vi "Debug Server First Launch.vi"(8 "error in (no error)":errorcluster, 11 "Debug Server in":refnum<class "Debug Server.lvclass">) -> (0 "error out":errorcluster, 3 "Debug Server out":refnum<class "Debug Server.lvclass">)   [LabVIEW 2017, in "Debug Server.lvclass"]
uses:
  Debug Server.lvclass
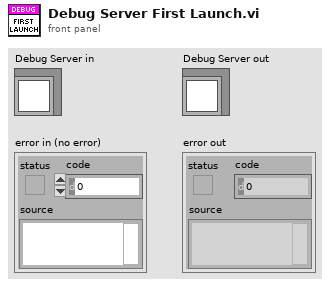
[diagram p1: front panel]
types:
  T1 = enum16{"open", "replace", "create", "open or create", "replace or create", "replace or create with confirmation"}
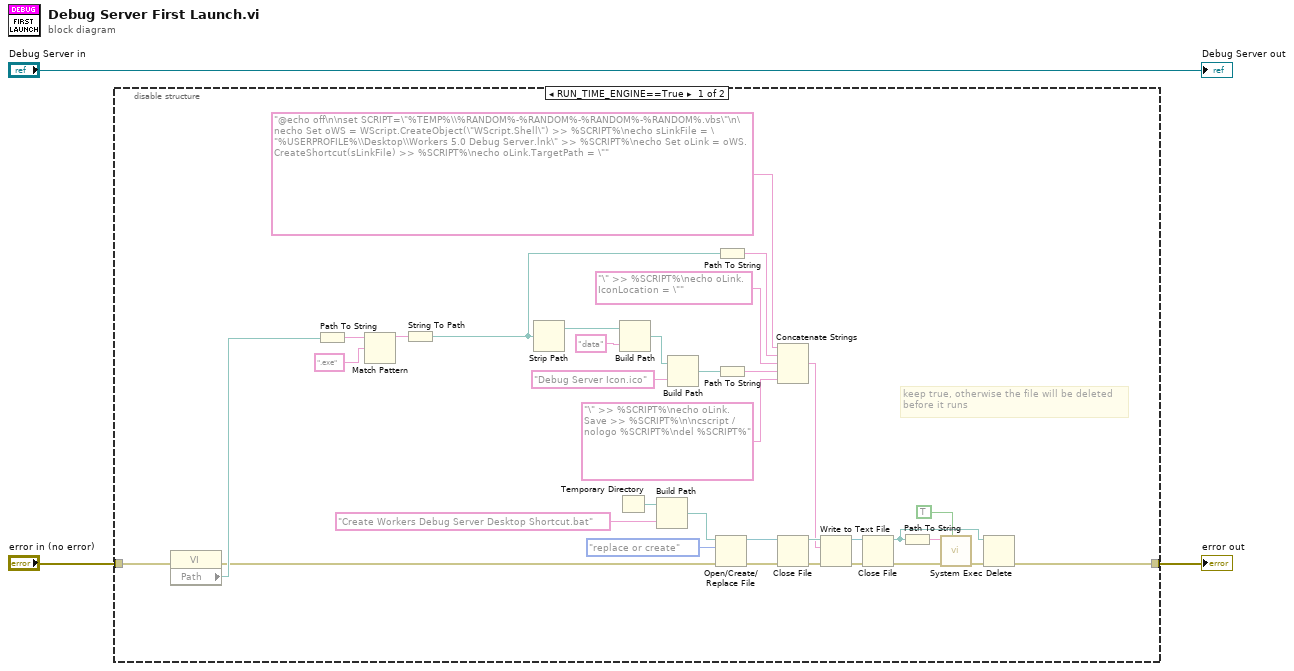
[diagram p0: block diagram]
diagram:
  n1 = disable-structure shown="RUN_TIME_ENGINE==True" {
    disable-tunnel: "error in (no error)" -> [w8 w38]
    disable-tunnel: [w7 w38] -> w1
    frame condition #0 {
      # "keep true, otherwise the file will be deleted\nbefore it runs"
      n2 = property class="VI"(error in=w8) -> (error out=w10:errorcluster, "Path"=w37:path)  [unwired: 1 in, 1 out]
      n3 = Path To String(path=w37) -> (string=w5:string)
      n4 = Match Pattern(string=w5, regular expression=".exe") -> (before substring=w6:string)  [unwired: 1 in, 3 out]
      n5 = String To Path(string=w6) -> (path=w31:path)
      n6 = Strip Path(path=w31) -> (stripped path=w33:path)  [unwired: 1 out]
      n7 = Temporary Directory() -> (w25:path)
      n8 = Build Path(base path=w33, name or relative path="data") -> (appended path=w30:path)
      n9 = Build Path(base path=w25, name or relative path="Create Workers Debug Server Desktop Shortcut.bat") -> (appended path=w24:path)
      n10 = Build Path(base path=w30, name or relative path="Debug Server Icon.ico") -> (appended path=w28:path)
      n11 = Open/Create/Replace File(file path (use dialog)=w24, error in=w10, operation (0:open)=T1."replace or create") -> (refnum out=w21:refnum<file>, error out=w22:errorcluster)  [unwired: 3 in, 1 out]
      n12 = Path To String(path=w31) -> (string=w36:string)
      n13 = Path To String(path=w28) -> (string=w27:string)
      n14 = Concatenate Strings("@echo off\n\nset SCRIPT=\"%TEMP%\\%RANDOM%-%RANDOM%-%RANDOM%-%RANDOM%.vbs\"\n\necho Set oWS = WScript.CreateObject(\"WScript.Shell\") >> %SCRIPT%\necho sLinkFile = \"%USERPROFILE%\\Desktop\\Workers 5.0 Debug Server.lnk\" >> %SCRIPT%\necho Set oLink = oWS.CreateShortcut(sLinkFile) >> %SCRIPT%\necho oLink.TargetPath = \"", w36, "\" >> %SCRIPT%\necho oLink.IconLocation = \"", w27, "\" >> %SCRIPT%\necho oLink.Save >> %SCRIPT%\n\ncscript /nologo %SCRIPT%\ndel %SCRIPT%") -> (w18:string)
      n15 = Close File(refnum=w21, error in=w22) -> (path=w19:path, error out=w20:errorcluster)
      n16 = Write to Text File(file (use dialog)=w19, text=w18, error in=w20) -> (refnum out=w16:refnum<file>, error out=w17:errorcluster)  [unwired: 1 in, 1 out]
      n17 = Close File(refnum=w16, error in=w17) -> (path=w11:path, error out=w14:errorcluster)
      n18 = Path To String(path=w11) -> (string=w12:string)
      n19 = call <vilib>:"System Exec.vi"("wait until completion? (T)"=TRUE, "error in (no error)"=w14, "command line"=w12) -> ("error out"=w13:errorcluster)  [unwired: 5 in, 3 out]
      n20 = Delete(path (use dialog)=w11, error in=w13) -> (error out=w7:errorcluster)  [unwired: 3 in, 2 out]
    }
    frame condition #1 (active) {
    }
  }
  "error out" <- w1
  "Debug Server out" <- "Debug Server in"
